vi "LINX - Blink + Measure -- SingleError.vi"() -> ()   [LabVIEW 2025]
doc: "Automatically blink and LED attached to a digital output channel of a LINX device."
uses:
  <vilib>/MakerHub/LINX/Public/Peripherals/Analog/Analog Read 1 Chan.vi
  <vilib>/MakerHub/LINX/Public/Peripherals/Digital/Digital Write 1 Chan.vi
  <vilib>/MakerHub/LINX/Public/Peripherals/Analog/Analog Read N Chans.vi
  <vilib>/MakerHub/LINX/Public/Peripherals/Digital/Digital Write N Chans.vi
  <vilib>/MakerHub/LINX/Private/Local IO/LinxAnalogRead.vi
  <vilib>/MakerHub/LINX/Public/Utilities/Check Channel.vi
  <vilib>/MakerHub/LINX/Private/Local IO/LinxDigitalWrite.vi
  <vilib>/MakerHub/LINX/Public/Utilities/Open Serial.vi
  <vilib>/MakerHub/LINX/Private/Utilties/Generate Error.vi
  <vilib>/MakerHub/LINX/LMH-LINX.lvlib
panel:
  in  "MeasStop":bool
  in  "milliseconds to wait":u32(slide) scale=50.0..1000.0
  in  "AI Channel":u8
  out "MeasLoop Rate (Hz)":u32
  out "Analog Data":dbl(graph)
  out "LED Value":bool
  in  "Digital Output Channel":u8=13
  in  "Serial Port":refnum<visa-resource-name>
  out "SrcLoop Rate (Hz)":u32
  in  "Stop Button":bool
  # "Circuit Schematic"
  # "LINX Device Settings"
  # "LED Value"
  # "LINX Device Settings"
  # "Analog Value"
  # "Blink (Serial Interface)\n\nThis example demonstrates how to blink an LED on a LINX device connected to \nthe host computer using USB / Serial.\n\nInstructions\n1. Select the Serial Port associated with the LINX Device.\n2. Select the Digital Pin connected to the LED.\n3. Click the Run Arrow."
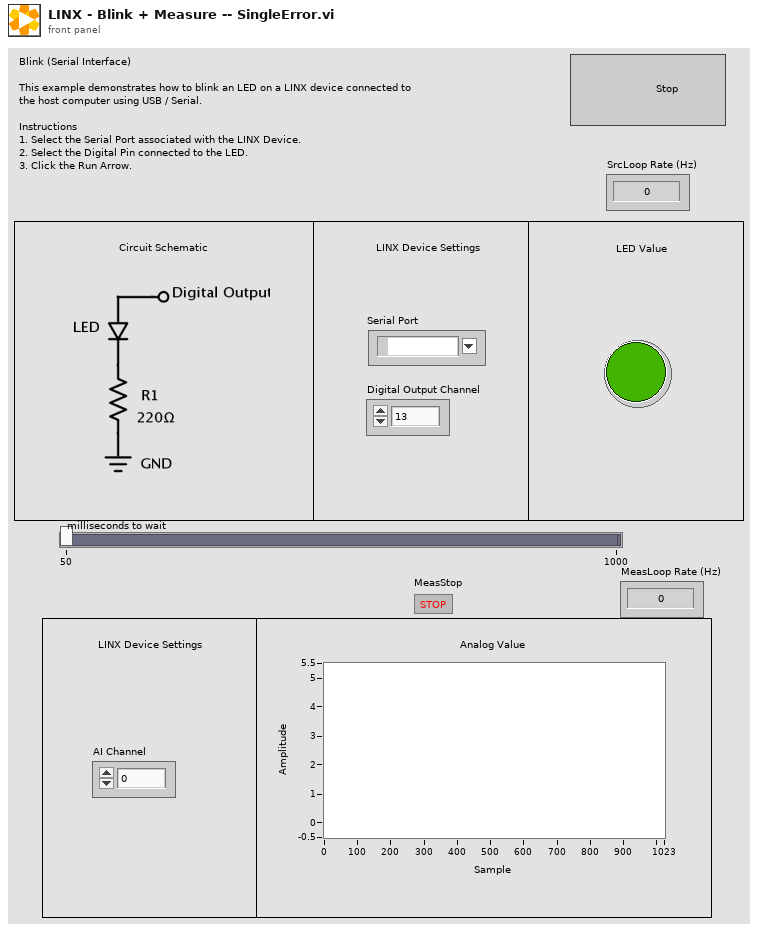
[diagram p1: front panel]
types:
  T1 = typedef "LMH-LINX.lvlib/LINX Ref.ctl" = cluster{"IO":T2, "Interface":T3, "LINX Device Config":T4}
  T2 = typedef "LMH-LINX.lvlib/Platform.ctl" = enum16{"Remote", "Local"}
  T3 = typedef "LMH-LINX.lvlib/Interface.ctl" = enum16{"Serial", "TCP"}
  T4 = typedef "LMH-LINX.lvlib/Device.lvlib/LINX Device Config.ctl" = cluster{"Interface":T3, "COM Port":refnum<visa-resource-name>, "TCP Configuration":T5, "Device Family":u8, "Device ID":u8, "Device Name":string, "TCP Ref":refnum<k5>, "Channels":T6}
  T5 = typedef "LMH-LINX.lvlib/Device.lvlib/TCP Config.ctl" = cluster{"IP Address":string, "Port":u16}
  T6 = typedef "LMH-LINX.lvlib/Channels.ctl" = cluster{"DI":u8[], "DO":u8[], "AI":u8[], "AO":u8[], "PWM":u8[], "QE":u8[], "UART":u8[], "I2C 2":u8[], "SPI":u8[], "CAN":u8[], "Servo":u8[], "AI Ref (V)":dbl, "AI Resolution (Bits)":u8, "AO Ref (V)":dbl, "AO Resolution (Bits)":u8}
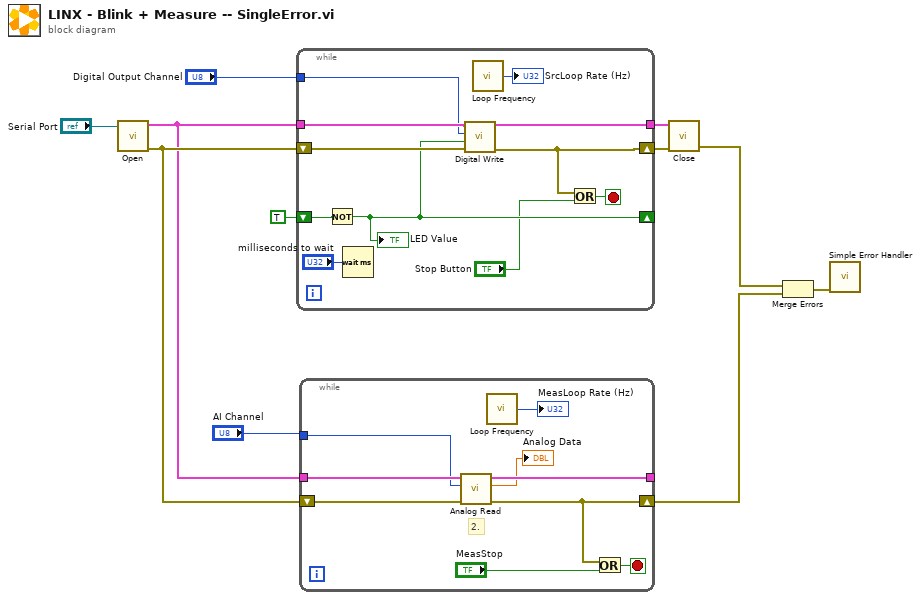
[diagram p0: block diagram]
diagram:
  n1 = call-poly <vilib>:"Open.vi"("Serial Port"="Serial Port") -> ("Error Out"=w6:errorcluster, "LINX Resource"=w5:T1)  [unwired: 8 in, 1 out]
  n2 = while {
    tunnel: w5 -> [w20]
    tunnel: [w19] -> w11
    shift-right: [w17] -> w1
    shift-left: w6 -> [w18]
    shift-right: [w14] -> _
    shift-left: TRUE -> [w15]
    tunnel: "Digital Output Channel" -> [w16]
    stop <- w22 stop-if-true
    n3 = Not(x=w15) -> (.not. x?=w14:bool)
    "LED Value" <- w14
    n4 = Wait (ms)(milliseconds to wait="milliseconds to wait") -> ()  [unwired: 1 out]
    n5 = call-poly <vilib>:"Digital Write.vi"("Error In"=w18, "Output Value"=w14, "DO Channel"=w16, "LINX Resource"=w20) -> ("Error Out"=w17:errorcluster, "LINX Resource"=w19:T1)  [unwired: 6 in]
    n6 = call <vilib>:"Loop Frequency.vi"() -> ("Loop Rate (Hz)"=→"SrcLoop Rate (Hz)":u32)
    n7 = Or(x=w17, y="Stop Button") -> (x .or. y?=w22:bool)
  }
  n8 = while {
    tunnel: w5 -> [w31]
    tunnel: [w29] -> _
    shift-right: [w27] -> w4
    shift-left: w6 -> [w30]
    tunnel: "AI Channel" -> [w26]
    stop <- w28 stop-if-true
    # "2."
    n9 = call-poly <vilib>:"Analog Read.vi"("Error In"=w30, "Analog Channel"=w26, "LINX Resource"=w31) -> ("Error Out"=w27:errorcluster, "Voltage"=→"Analog Data":dbl, "LINX Resource"=w29:T1)  [unwired: 5 in, 1 out]
    n10 = call <vilib>:"Loop Frequency.vi"() -> ("Loop Rate (Hz)"=→"MeasLoop Rate (Hz)":u32)
    n11 = Or(x=w27, y="MeasStop") -> (x .or. y?=w28:bool)
  }
  n12 = call <vilib>:"Close.vi"("Error In"=w1, "LINX Resource"=w11) -> ("Error Out"=w2:errorcluster)  [unwired: 9 in]
  n13 = Merge Errors(w2, w4) -> (w3:errorcluster)
  n14 = call <vilib>:"Simple Error Handler.vi"("error in (no error)"=w3) -> ()  [unwired: 4 in, 5 out]
